vi "Get Bitfile Scalars.vi"(8 "error in (no error)":errorcluster, 11 "fpga addon refnum in":T2=18446744073709551615 format="%.0x") -> (0 "error out":errorcluster, 2 "bitfile scalars out":T1[](array[typedef]), 3 "fpga addon refnum out":T2=18446744073709551615 format="%.0x")   [LabVIEW 2018, in "Scripting API.lvlib"]
uses:
  Scripting API.lvlib
  <vilib>/NI Veristand/Custom Device API/Custom Device Item Ref.ctl
  TypeDefs/Output Scalar Data.ctl
  <vilib>/NI Veristand/Custom Device API/Custom Device API.lvlib
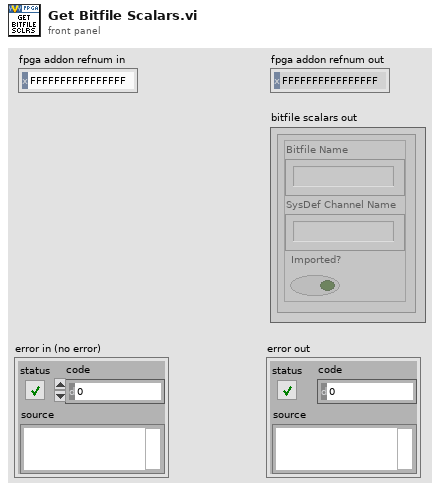
[diagram p1: front panel]
types:
  T1 = typedef "Scripting API.lvlib/Output Scalar Data.ctl" = cluster{"Bitfile Name":string, "SysDef Channel Name":string, "Imported?":bool}
  T2 = typedef "Custom Device API.lvlib/Custom Device Item Ref.ctl" = u64
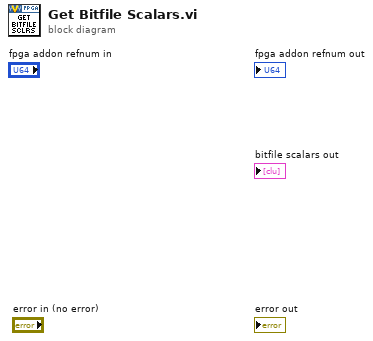
[diagram p0: block diagram]
diagram:
